vi "Append Conditional Ring Text.vi"(0 "Append":bool, 1 "New Chans":cluster{string[]}[](array[cluster]), 2 "New Params":cluster{string[]}[](array[cluster]), 3 "New States":string[](array[string]), 5 "States In":string[](array[string]), 7 "Chans In":cluster{string[]}[](array[cluster]), 9 "Params In":cluster{"Properties":string[]}[][](array[cluster])) -> (6 "States Out":string[](array[string]), 8 "Chans Out":cluster{string[]}[](array[cluster]), 10 "Params Out":cluster{"Properties":string[]}[][](array[cluster]))   [LabVIEW 2020, in "Parameters.lvclass"]
uses:
  Parameters.lvclass
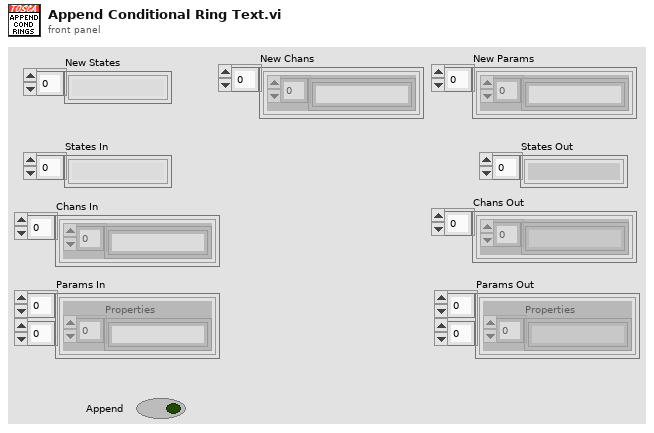
[diagram p1: front panel]
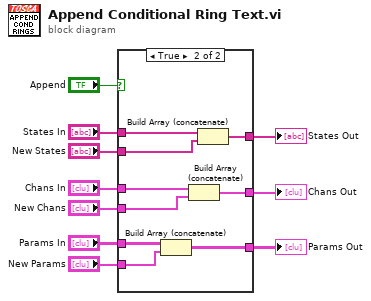
[diagram p0: block diagram]
diagram:
  n1 = case shown="True" "Append" {
    tunnel: "States In" -> [w13 w22]
    tunnel: "Chans In" -> [w12 w21]
    tunnel: "Params In" -> [w11 w20]
    tunnel: [w13 w19] -> w10
    tunnel: "New States" -> [_ w18]
    tunnel: [w12 w17] -> w9
    tunnel: "New Chans" -> [_ w16]
    tunnel: [w11 w15] -> w8
    tunnel: "New Params" -> [_ w14]
    frame False {
    }
    frame True {
      n2 = Build Array (concatenate)(w20, w14) -> (w15:cluster{"Properties":string[]}[][])
      n3 = Build Array (concatenate)(w21, w16) -> (w17:cluster{string[]}[])
      n4 = Build Array (concatenate)(w22, w18) -> (w19:string[])
    }
  }
  "States Out" <- w10
  "Chans Out" <- w9
  "Params Out" <- w8
